vi "DSFLSHdll.vi"(8 "error in (no error)":errorcluster, 11 "FLSH Inputs":T1={"t"=0.0, "p"=0.0, "e"=0.0, "h"=0.0, "s"=0.0, "q"=0.0, "z"=[0.0, 0.0, 0.0, 0.0, 0.0, 0.0, 0.0, 0.0, 0.0, 0.0, 0.0, 0.0, 0.0, 0.0, 0.0, 0.0, 0.0, 0.0, 0.0, 0.0], "kq"=0, "kr"=0, "D"=0.0}) -> (0 "error out":errorcluster, 3 "FLSH Outputs":T2)   [LabVIEW 2016]
doc: "GENERAL FLASH SUBROUTINES\n\nflash calculation given two independent variables and bulk composition\n\nThese routines accept both single-phase and two-phase states as the\ninput; if the phase is known, the specialized routines are faster\n\nINPUTS -- two of the following as indicated by the first two letters of the subroutine name:\n t--temperature [K]\n p--pressure [kPa]\n e--internal energy [J/mol]\n h--enthalpy [J/mol]\n s--entropy [[J/mol-K]\n q--vapor quality [basis specified by kq]\n q = 0 indicates saturated liquid\n q = 1 indicates saturated vapor\n q < 0 or q > 1 are not allowed and will result in warning\n\n additional input--required for all routines\n z--overall (bulk) composition [array of mol frac]\n\n additional input--only for TQFLSH and PQFLSH\n kq--flag specifying units for input quality\n kq = 1 quality on MOLAR basis [moles vapor/total moles]\n kq = 2 quality on MASS basis [mass vapor/total mass]\n\n additional input--only for THFLSH, TSFLSH, and TEFLSH\n kr--flag specifying desired root for multi-valued inputs:\n 1 = return lower density root\n 2 = return higher density root\n\nOUTPUTS -- one, two, or all of the following, depending on the inputs:\n t--temperature [K]\n p--pressure [kPa]\n D--overall (bulk) molar density [mol/L]\n\n additional outputs--common to all routines\n Dl--molar density [mol/L] of the liquid phase\n Dv--molar density [mol/L] of the vapor phase\n if only one phase is present, Dl = Dv = D\n x--composition of liquid phase [array of mol frac]\n y--composition of vapor phase [array of mol frac]\n if only one phase is present, x = y = z\n\n additional output--common to all routines except TQFLSH and PQFLSH\n q--vapor quality on a MOLAR basis [moles vapor/total moles]\n q < 0 indicates subcooled (compressed) liquid\n q = 0 indicates saturated liquid\n q = 1 indicates saturated vapor\n q > 1 indicates superheated vapor\n q = 998 superheated vapor, but quality not defined (in most situations, t > Tc)\n q = 999 indicates supercritical state (t > Tc) and (p > Pc)\n\n additional outputs--common to all routines, except that input quantities are not repeated\n e--overall (bulk) internal energy [J/mol]\n h--overall (bulk) enthalpy [J/mol]\n s--overall (bulk) entropy [J/mol-K]\n Cv--isochoric (constant V) heat capacity [J/mol-K]\n Cp--isobaric (constant p) heat capacity [J/mol-K]\n w--speed of sound [m/s]\n cp, w are not defined for 2-phase states in such cases, a flag = -9.99998d6 is returned\n ierr--error flag: 0 = all inputs within limits\n <>0 = one or more inputs outside limits:\n -1 = 1.5*tmax > t > tmax\n 1 = t < tmin or t > 1.5*tmax\n 2 = D > Dmax or D < 0\n -4 = 2*pmax > p > pmax\n 4 = p < 0 or p > 2*pmax\n 8 = component composition < 0 or > 1\n and/or composition sum < 0 or > 1\n 16 = p>pmelt\n -16 = t<ttrp (important for water)\n if multiple inputs are outside limits, ierr = abs[sum(ierr)]\n with the sign determined by the most severe excursion\n (ierr > 0 indicate an error--calculations not possible,\n ierr < 0 indicate a warning--results may be questionable)\n herr--error string (character*255 variable if ierr<>0)\n herr_length-- length of variable herr (default: 255)"
uses:
  Ctl/FLSH_Outputs.ctl
  Ctl/FLSH_Inputs.ctl
  REFPROP.DLL
panel:
  # "REFPROP-DSFLSHdll.vi"
  # "subroutine DSFLSHdll(D, s, z, t, p, Dl, Dv, x, y, q, e, h, Cv, Cp, w, ierr, herr, herr_length)"
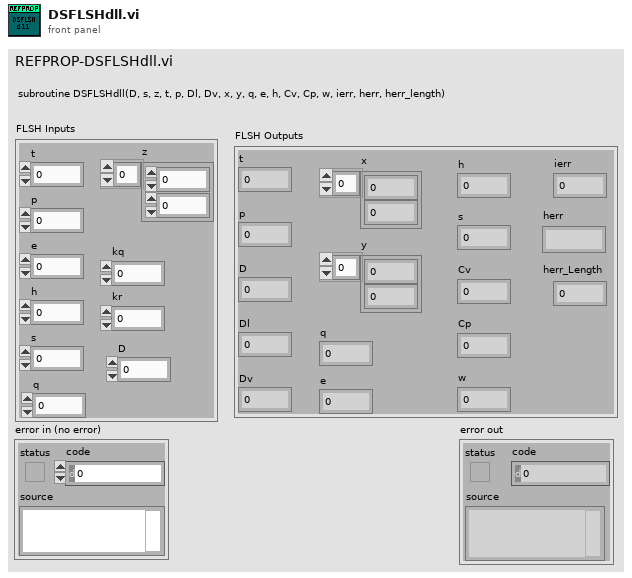
[diagram p1: front panel]
types:
  T1 = typedef "FLSH_Inputs.ctl" = cluster{"t":dbl, "p":dbl, "e":dbl, "h":dbl, "s":dbl, "q":dbl, "z":dbl[], "kq":i32, "kr":i32, "D":dbl}
  T2 = typedef "FLSH_Outputs.ctl" = cluster{"t":dbl, "p":dbl, "D":dbl, "Dl":dbl, "Dv":dbl, "x":dbl[], "y":dbl[], "q":dbl, "e":dbl, "h":dbl, "s":dbl, "Cv":dbl, "Cp":dbl, "w":dbl, "ierr":i32, "herr":string, "herr_Length":i32}
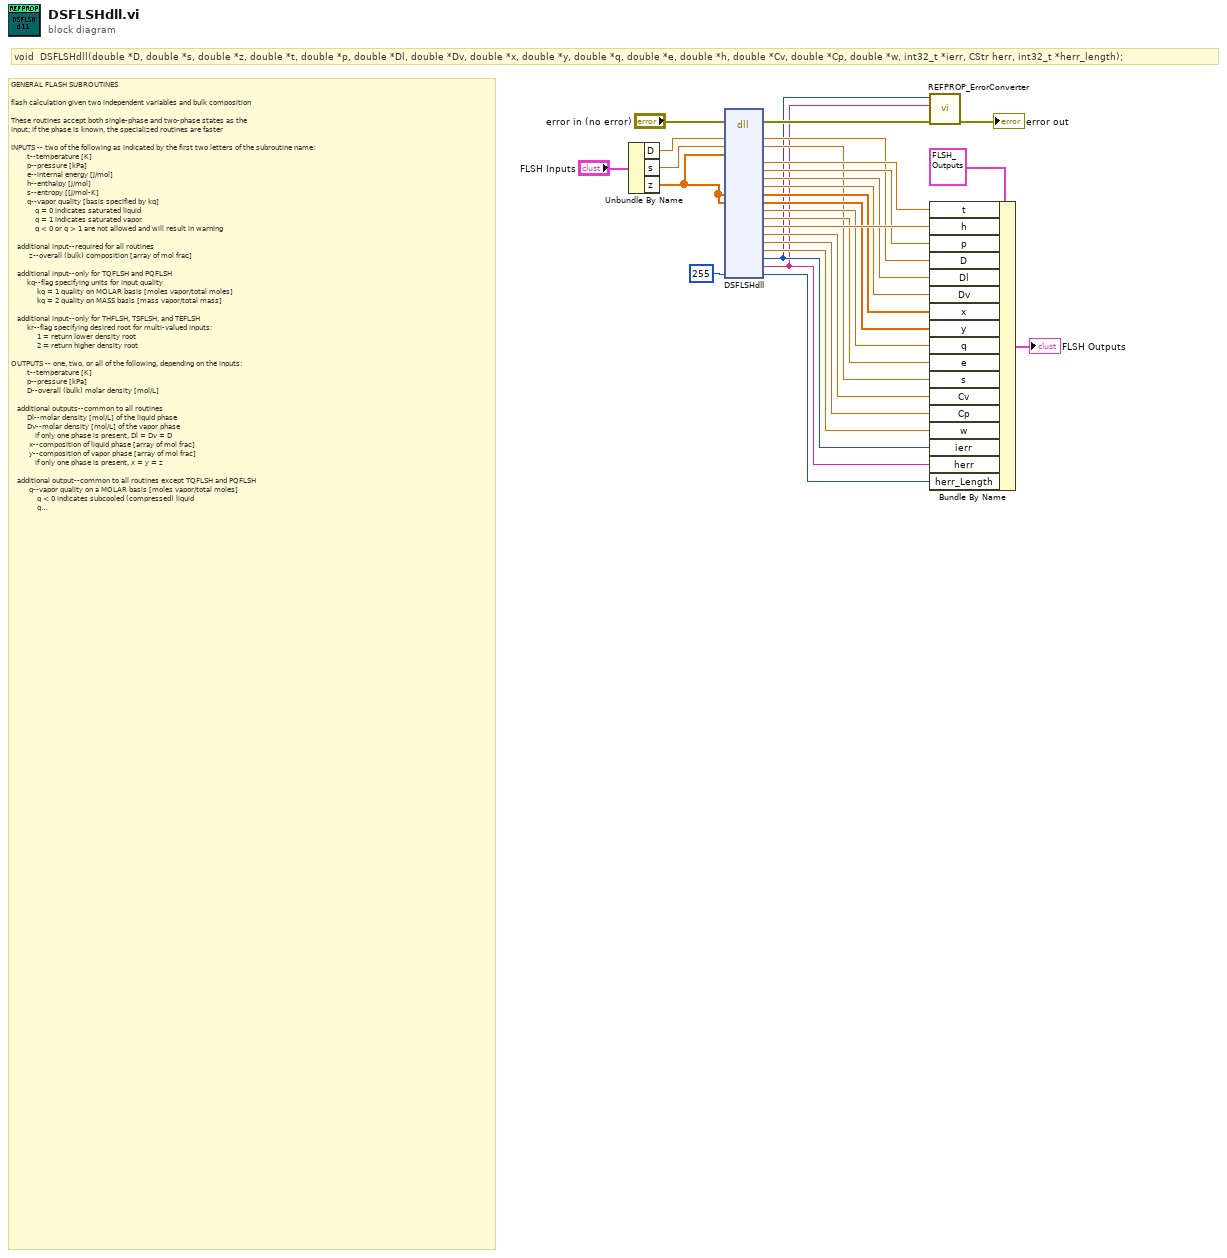
[diagram p0: block diagram]
diagram:
  # "GENERAL FLASH SUBROUTINES\n\nflash calculation given two independent variables and bulk composition\n\nThese routines accept both single-phase and two-phase states as the\ninput; if the phase is known, the specialized routines are faster\n\nINPUTS -- two of the following as indicated by the first two letters of the subroutine name:\n        t--temperature [K]\n        p--pressure [kPa]\n        e--internal energy [J/mol]\n        h--enthalpy [J/mol]\n        s--entropy [[J/mol-K]\n        q--vapor quality [basis specified by kq]\n            q = 0 indicates saturated liquid\n            q = 1 indicates saturated vapor\n            q < 0 or q > 1 are not allowed and will result in warning\n\n   additional input--required for all routines\n         z--overall (bulk) composition [array of mol frac]\n\n   additional input--only for TQFLSH and PQFLSH\n        kq--flag specifying units for input quality\n             kq = 1 quality on MOLAR basis [moles vapor/total moles]\n             kq = 2 quality on MASS basis [mass vapor/total mass]\n\n   additional input--only for THFLSH, TSFLSH, and TEFLSH\n        kr--flag specifying desired root for multi-valued inputs:\n             1 = return lower density root\n             2 = return higher density root\n\nOUTPUTS -- one, two, or all of the following, depending on the inputs:\n        t--temperature [K]\n        p--pressure [kPa]\n        D--overall (bulk) molar density [mol/L]\n\n   additional outputs--common to all routines\n        Dl--molar density [mol/L] of the liquid phase\n        Dv--molar density [mol/L] of the vapor phase\n            if only one phase is present, Dl = Dv = D\n         x--composition of liquid phase [array of mol frac]\n         y--composition of vapor phase [array of mol frac]\n            if only one phase is present, x = y = z\n\n   additional output--common to all routines except TQFLSH and PQFLSH\n         q--vapor quality on a MOLAR basis [moles vapor/total moles]\n             q < 0 indicates subcooled (compressed) liquid\n             q = 0 indicates saturated liquid\n             q = 1 indicates saturated vapor\n             q > 1 indicates superheated vapor\n             q = 998 superheated vapor, but quality not defined (in most situations, t > Tc)\n             q = 999 indicates supercritical state (t > Tc) and (p > Pc)\n\n   additional outputs--common to all routines, except that input quantities are not repeated\n         e--overall (bulk) internal energy [J/mol]\n         h--overall (bulk) enthalpy [J/mol]\n         s--overall (bulk) entropy [J/mol-K]\n         Cv--isochoric (constant V) heat capacity [J/mol-K]\n         Cp--isobaric (constant p) heat capacity [J/mol-K]\n         w--speed of sound [m/s]\n             cp, w are not defined for 2-phase states in such cases, a flag = -9.99998d6 is returned\n         ierr--error flag:  0 = all inputs within limits\n                      <>0 = one or more inputs outside limits:\n                       -1 = 1.5*tmax > t > tmax\n                        1 = t < tmin or t > 1.5*tmax\n                        2 = D > Dmax or D < 0\n                       -4 = 2*pmax > p > pmax\n                        4 = p < 0 or p > 2*pmax\n                        8 = component composition < 0 or > 1\n                            and/or composition sum < 0 or > 1\n                       16 = p>pmelt\n                      -16 = t<ttrp (important for water)\n           if multiple inputs are outside limits, ierr = abs[sum(ierr)]\n           with the sign determined by the most severe excursion\n           (ierr > 0 indicate an error--calculations not possible,\n            ierr < 0 indicate a warning--results may be questionable)\n         herr--error string (character*255 variable if ierr<>0)\n         herr_length-- length of variable herr (default: 255)"
  # "void  DSFLSHdll(double *D, double *s, double *z, double *t, double *p, double *Dl, double *Dv, double *x, double *y, double *q, double *e, double *h, double *Cv, double *Cp, double *w, int32_t *ierr, CStr herr, int32_t *herr_length);"
  n1 = Unbundle By Name("FLSH Inputs") -> ("D"=w20:dbl, "s"=w19:dbl, "z"=w1:dbl[])
  n2 = dll-call lib="C:/Program Files (x86)/REFPROP/refprop.*" fn="DSFLSHdll"(error in="error in (no error)", "D"=w20, "s"=w19, "z"=w1, "x"=w1, "y"=w1, "herr_length"=255 ("ln")) -> (error out=w25:errorcluster, "D"=w15:dbl, "s"=w8:dbl, "t"=w18:dbl, "p"=w16:dbl, "Dl"=w14:dbl, "Dv"=w13:dbl, "x"=w12:dbl[], "y"=w11:dbl[], "q"=w10:dbl, "e"=w9:dbl, "h"=w17:dbl, "Cv"=w7:dbl, "Cp"=w6:dbl, "w"=w5:dbl, "ierr"=w4:i32, "herr"=w3:string, "herr_length"=w2:i32)  [unwired: 16 in, 1 out]
  n3 = call "REFPROP_ErrorConverter.vi"("error in (no error)"=w25, "Error Message"=w3, "Error Code"=w4) -> ("error out"=→"error out":errorcluster)  [unwired: 8 in]
  n4 = Bundle By Name(cluster=T2 {"t"=0.0, "p"=0.0, "D"=0.0, "Dl"=0.0, "Dv"=0.0, "x"=[0.0, 0.0, 0.0, 0.0, 0.0, 0.0, 0.0, 0.0, 0.0, 0.0, 0.0, 0.0, 0.0, 0.0, 0.0, 0.0, 0.0, 0.0, 0.0, 0.0], "y"=[0.0, 0.0, 0.0, 0.0, 0.0, 0.0, 0.0, 0.0, 0.0, 0.0, 0.0, 0.0, 0.0, 0.0, 0.0, 0.0, 0.0, 0.0, 0.0, 0.0], "q"=0.0, "e"=0.0, "h"=0.0, "s"=0.0, "Cv"=0.0, "Cp"=0.0, "w"=0.0, "ierr"=0, "herr"="", "herr_Length"=0} ("FLSH Outputs 2"), "t"=w18, "h"=w17, "p"=w16, "D"=w15, "Dl"=w14, "Dv"=w13, "x"=w12, "y"=w11, "q"=w10, "e"=w9, "s"=w8, "Cv"=w7, "Cp"=w6, "w"=w5, "ierr"=w4, "herr"=w3, "herr_Length"=w2) -> (→"FLSH Outputs":T2)
